vi "DUAL GAUGE-RW Unit.vi"(7 "W/R":bool, 8 "Fehler (Eingang)":errorcluster, 9 "Unit Set":i8(ring) items=["mbar / bar", "Torr", "Pascal"], 11 "Referenz in":refnum<visa-resource-name>) -> (0 "Cluster (Ausgang)":errorcluster, 1 "Unit Get":i8(ring) items=["mbar / bar", "Torr", "Pascal"], 3 "Referenz out":refnum<visa-resource-name>)   [LabVIEW 2017, in "Dual Gauge.lvlib"]
uses:
  <userlib>/Dual Gauge/Dual Gauge.lvlib
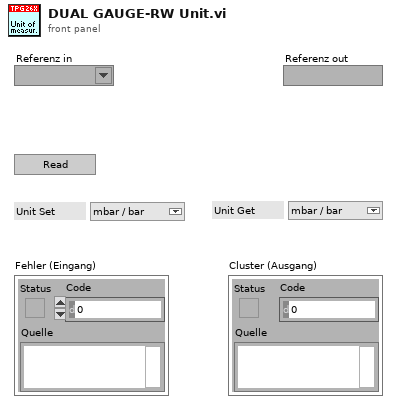
[diagram p1: front panel]
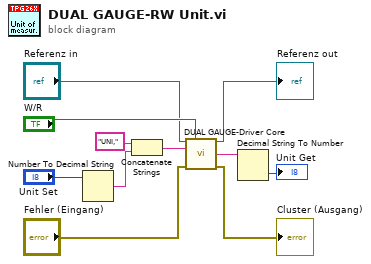
[diagram p0: block diagram]
diagram:
  n1 = Number To Decimal String(number="Unit Set") -> (decimal integer string=w7:string)  [unwired: 1 in]
  n2 = Concatenate Strings("UNI,", w7) -> (w5:string)
  n3 = call <userlib>:"DUAL GAUGE-Driver Core.vi"("Referenz in"="Referenz in", "Write/Read"="W/R", "Command"=w5, "Fehler (Eingang)"="Fehler (Eingang)") -> ("Referenz out"=→"Referenz out":refnum<visa-resource-name>, "String Out"=w6:string, "Cluster (Ausgang)"=→"Cluster (Ausgang)":errorcluster)  [unwired: 9 in]
  n4 = Decimal String To Number(string=w6) -> (number=→"Unit Get":i32)  [unwired: 2 in, 1 out]
